vi "File4.vi"(2 "Pocet ignorovanych vzorku":dbl, 3 "X":dbl[](array[numeric]), 4 "dt":dbl, 5 "Y":dbl[](array[numeric])) -> (0 "Indexy pruchodu nulou":i32[](array[numeric]), 1 "XY Graph":cluster{"Array":dbl[], "Y":dbl[]}(graph))   [LabVIEW 2019]
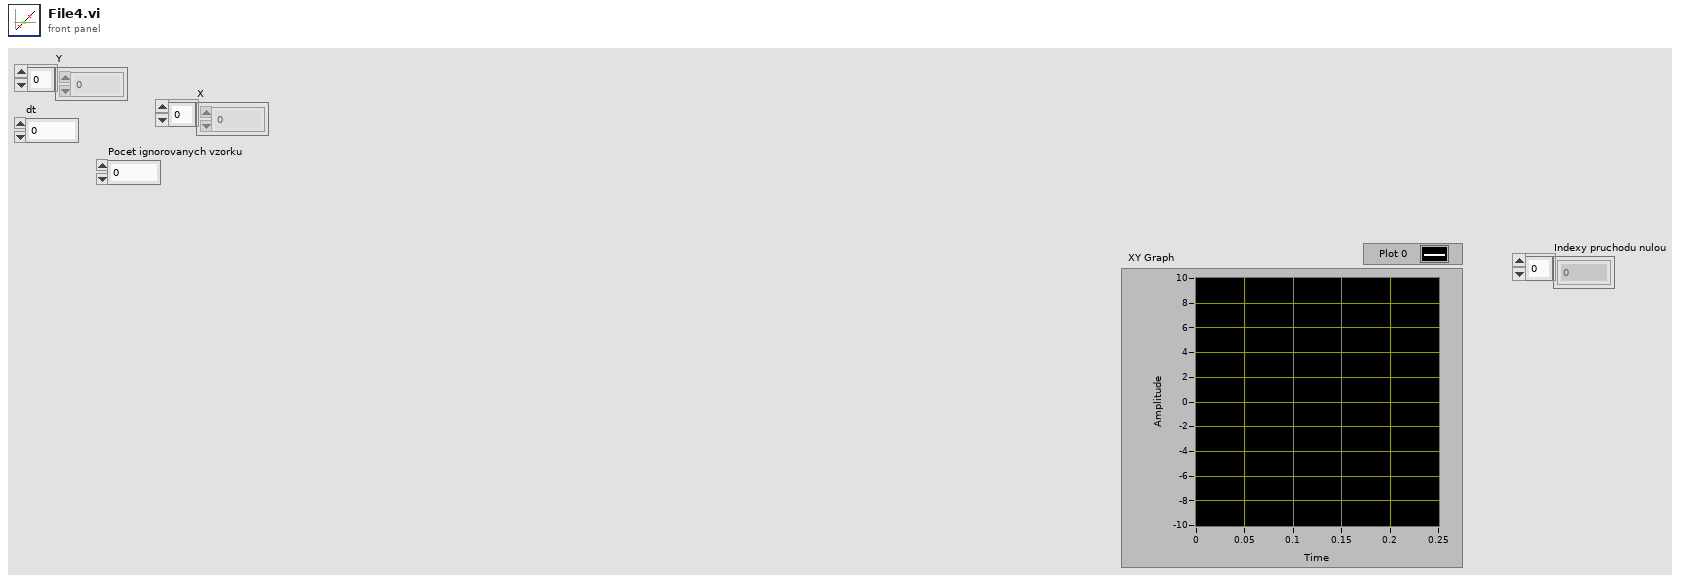
[diagram p1: front panel]
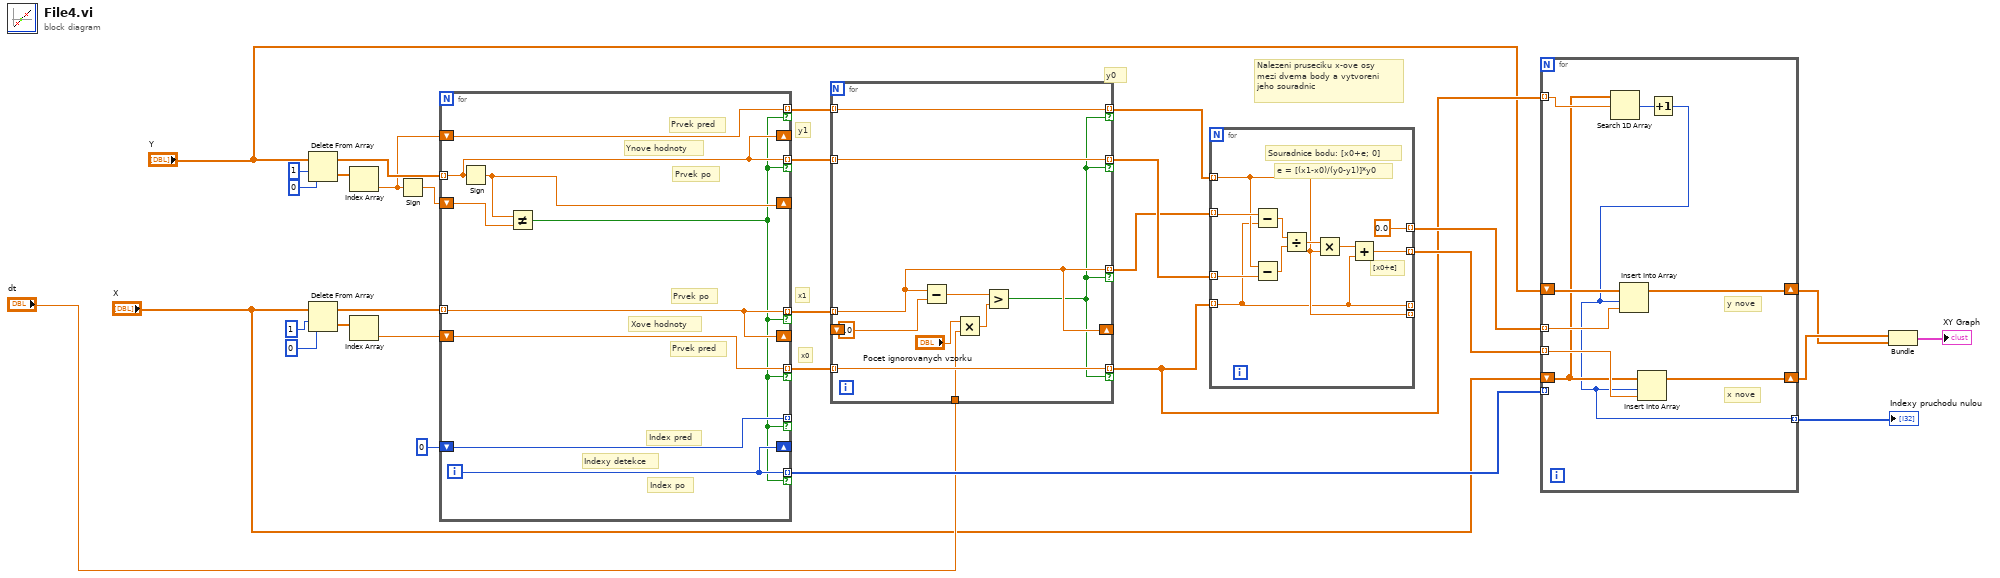
[diagram p0: block diagram]
diagram:
  # "Nalezeni pruseciku x-ove osy\nmezi dvema body a vytvoreni\njeho souradnic"
  # "x0"
  # "y0"
  # "x1"
  # "y1"
  n1 = Delete From Array(array="Y", length=1, index=0) -> (deleted portion=w29:dbl[], array with subset deleted=w26:dbl[])
  n2 = Delete From Array(array="X", length=1, index=0) -> (deleted portion=w23:dbl[], array with subset deleted=w25:dbl[])
  n3 = Index Array(array=w29) -> (element=w21:dbl)  [unwired: 1 in]
  n4 = Index Array(array=w23) -> (element=w22:dbl)  [unwired: 1 in]
  n5 = Sign(1:w21) -> (0:w24:dbl)
  n6 = for {
    tunnel: w26 -> [w35] mode=indexing
    tunnel: w25 -> [w38] mode=indexing
    shift-right: [w39] -> _
    shift-left: w24 -> [w40]
    shift-right: [w38] -> _
    shift-left: w22 -> [w37]
    tunnel: [w38] -> w10 mode=indexing if=w32
    tunnel: [w37] -> w9 mode=indexing if=w32
    shift-right: [w35] -> _
    shift-left: w21 -> [w36]
    tunnel: [w36] -> w12 mode=indexing if=w32
    tunnel: [w35] -> w11 mode=indexing if=w32
    shift-right: [w34] -> _
    shift-left: 0 -> [w33]
    tunnel: [w34] -> w17 mode=indexing if=w32
    tunnel: [w33] -> _ mode=indexing if=w32
    i -> [w34]
    # "Indexy detekce"
    # "Index po"
    # "Index pred"
    # "Ynove hodnoty"
    # "Prvek po"
    # "Prvek pred"
    # "Xove hodnoty"
    # "Prvek pred"
    # "Prvek po"
    n7 = Sign(1:w35) -> (0:w39:dbl)
    n8 = Not Equal?(x=w39, y=w40) -> (x != y?=w32:bool)
  }
  n9 = for {
    tunnel: w12 -> [w46] mode=indexing
    tunnel: w11 -> [w47] mode=indexing
    tunnel: w10 -> [w45] mode=indexing
    tunnel: w9 -> [w48] mode=indexing
    shift-right: [w45] -> _
    shift-left: 0.0 -> [w50]
    tunnel: [w45] -> w5 mode=indexing if=w44
    tunnel: [w48] -> w4 mode=indexing if=w44
    tunnel: [w47] -> w6 mode=indexing if=w44
    tunnel: [w46] -> w7 mode=indexing if=w44
    tunnel: "dt" -> [w42]
    n10 = Subtract(x=w45, y=w50) -> (x-y=w49:dbl)
    n11 = Multiply(x="Pocet ignorovanych vzorku", y=w42) -> (x*y=w41:dbl)
    n12 = Greater?(x=w49, y=w41) -> (0:w44:bool)
  }
  n13 = for {
    tunnel: [w52] -> _ mode=indexing
    tunnel: w4 -> [w52] mode=indexing
    tunnel: [w56] -> _ mode=indexing
    tunnel: w7 -> [w56] mode=indexing
    tunnel: w5 -> [w57] mode=indexing
    tunnel: w6 -> [w55] mode=indexing
    tunnel: [w54] -> w18 mode=indexing
    tunnel: [0.0] -> w19 mode=indexing
    # "[x0+e]"
    # "e = [(x1-x0)/(y0-y1)]*y0"
    # "Souradnice bodu: [x0+e; 0]"
    n14 = Subtract(x=w57, y=w52) -> (x-y=w59:dbl)
    n15 = Subtract(x=w56, y=w55) -> (x-y=w58:dbl)
    n16 = Divide(x=w59, y=w58) -> (x/y=w60:dbl)
    n17 = Multiply(x=w60, y=w56) -> (x*y=w53:dbl)
    n18 = Add(x=w53, y=w52) -> (x+y=w54:dbl)
  }
  n19 = for {
    tunnel: w17 -> [_] mode=indexing
    tunnel: w18 -> [w68] mode=indexing
    tunnel: w19 -> [w69] mode=indexing
    shift-right: [w67] -> w15
    shift-left: "Y" -> [w65]
    shift-right: [w66] -> w16
    shift-left: "X" -> [w63]
    tunnel: [w61] -> w13 mode=indexing
    tunnel: w4 -> [w64] mode=indexing
    # "x nove"
    # "y nove"
    n20 = Search 1D Array(1D array=w63, element=w64) -> (index of element=w62:i32)  [unwired: 1 in]
    n21 = Increment(x=w62) -> (x+1=w61:i32)
    n22 = Insert Into Array(array=w65, index=w61, new element=w69) -> (w67:dbl[])
    n23 = Insert Into Array(array=w63, index=w61, new element=w68) -> (w66:dbl[])
  }
  "Indexy pruchodu nulou" <- w13
  n24 = Bundle("X"=w16, "Y"=w15) -> (→"XY Graph":cluster{"X":dbl[], "Y":dbl[]})  [unwired: 1 in]
